vi "Update Subscription.vi"(8 "error in (no error)":errorcluster, 10 "Topic Subscription":T1, 11 "Client ID":string) -> (0 "error out":errorcluster)   [LabVIEW 2013, in "MQTT Server.lvlib" / "StoredSessions.lvclass"]
uses:
  StoredSessions.lvclass
  <vilib>/LabVIEW Open Source Project/MQTT Control Packets/Control Packets/SUBSCRIBE/Topic Subscription -- cluster.ctl
  <vilib>/LabVIEW Open Source Project/MQTT Control Packets/Control Packets/ControlPacket/QualityOfService -- enum.ctl
  Session State -- cluster.ctl
  <vilib>/LabVIEW Open Source Project/MQTT Control Packets/Control Packets/ControlPacket/ControlPacket.lvclass
  <vilib>/LabVIEW Open Source Project/MQTT Control Packets/Control Packets/SUBSCRIBE/SUBSCRIBE.lvclass
  Subscription/Subscription.lvclass
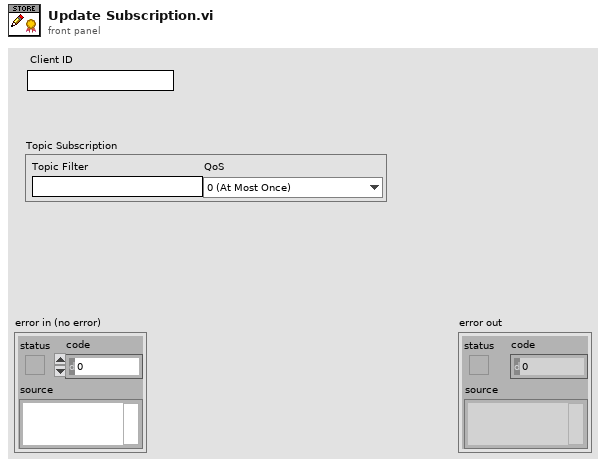
[diagram p1: front panel]
types:
  T1 = typedef "MQTT_Control_Packets.lvlib/SUBSCRIBE.lvclass/Topic Subscription -- cluster.ctl" = cluster{"Topic Filter":string, "QoS":T2}
  T2 = typedef "MQTT_Control_Packets.lvlib/ControlPacket.lvclass/QualityOfService -- enum.ctl" = enum16{"0 (At Most Once)", "1 (At Least Once)", "2 (Exactly Once)"}
  T3 = typedef "MQTT Server.lvlib/StoredSessions.lvclass/Session State -- cluster.ctl" = cluster{"Client ID":string, "Subscriptions":T1[], "PUBREC":u16[]}
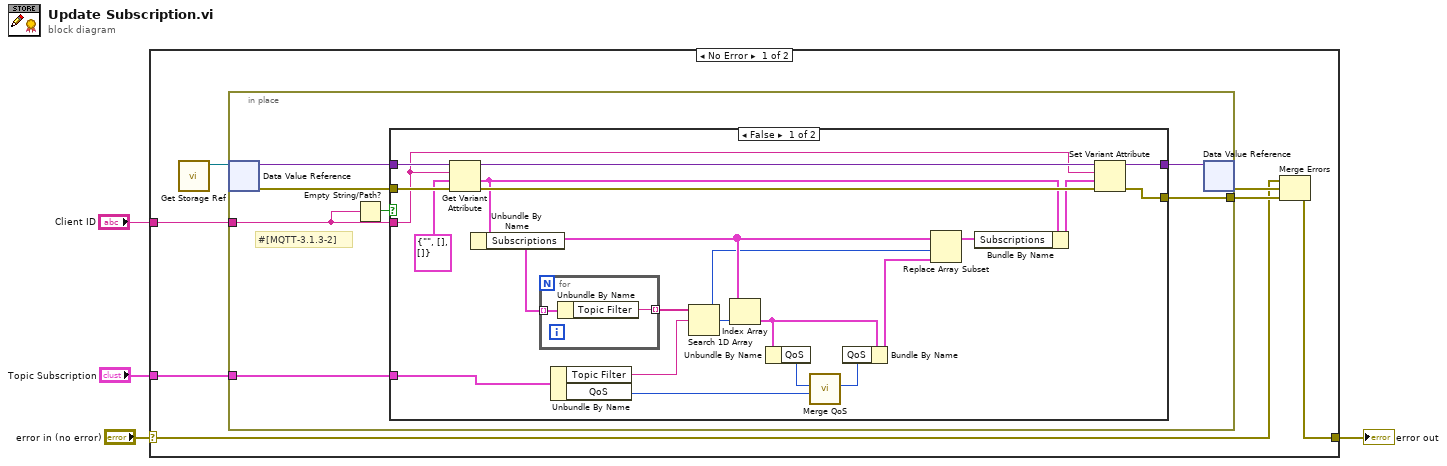
[diagram p0: block diagram]
diagram:
  n1 = case shown="No Error" "error in (no error)" {
    selector: "error in (no error)" -> [w7 w44]
    tunnel: [w6 w44] -> w3
    tunnel: "Topic Subscription" -> [w10 _]
    tunnel: "Client ID" -> [w5 _]
    frame No Error {
      n2 = call "Get Storage Ref.vi"() -> ("Storage"=w11:refnum<data-value>)  [unwired: 11 in]
      n3 = in-place {
        in-place-border: w10 -> [w12]
        in-place-border: [w16] -> w9
        in-place-border: w5 -> [w13]
        # "#[MQTT-3.1.3-2]"
        n4 = in-place-dvr #1(w11) -> (w18:variant, w15:errorcluster)
        n5 = Empty String/Path?(string/path=w13) -> (empty?=w14:bool)
        n6 = case shown="False" w14 {
          tunnel: w18 -> [w39 w43]
          tunnel: [w36 w43] -> w17
          tunnel: [w33 w42] -> w16
          tunnel: w15 -> [w38 w42]
          tunnel: w13 -> [w32 _]
          tunnel: w12 -> [w29 _]
          frame False {
            n7 = Get Variant Attribute(Variant=w39, name=w32, default value (empty Variant)=T3 {"Client ID"="", "Subscriptions"=[], "PUBREC"=[]} ("Stored Session"), error in=w38) -> (duplicate Variant=w37:variant, value=w31:T3, error out=w34:errorcluster)  [unwired: 1 out]
            n8 = Unbundle By Name(w31) -> ("Subscriptions"=w25:T1[])
            n9 = for {
              tunnel: w25 -> [w41] mode=indexing
              tunnel: [w40] -> w28 mode=indexing
              n10 = Unbundle By Name(w41) -> ("Topic Filter"=w40:string)
            }
            n11 = Unbundle By Name(w29) -> ("Topic Filter"=w27:string, "QoS"=w20:T2)
            n12 = Search 1D Array(1D array=w28, element=w27) -> (index of element=w24:i32)  [unwired: 1 in]
            n13 = Index Array(array=w25, index=w24) -> (element=w23:T1)
            n14 = Unbundle By Name(w23) -> ("QoS"=w21:T2)
            n15 = call "Merge QoS.vi"("Subscription QoS"=w20, "Message QoS"=w21) -> ("Highest QoS"=w19:T2)  [unwired: 9 in]
            n16 = Bundle By Name(cluster=w23, "QoS"=w19) -> (w22:T1)
            n17 = Replace Array Subset(array=w25, new element=w22, index=w24) -> (w26:T1[])
            n18 = Bundle By Name(cluster=w31, "Subscriptions"=w26) -> (w30:T3)
            n19 = Set Variant Attribute(Variant=w37, name=w32, value=w30, error in=w34) -> (Variant out=w36:variant, error out=w33:errorcluster)  [unwired: 1 out]
          }
          frame True {
          }
        }
        n20 = in-place-dvr #1(w17) -> (w8:errorcluster)  [unwired: 1 out]
      }
      n21 = Merge Errors(w7, w8, w9) -> (w6:errorcluster)
    }
    frame Error {
    }
  }
  "error out" <- w3
